vi "Manual_control.vi"(3 "Movement 2":T1={"Achsen-Wahl (X)"=36, "Richtung (vEw)"=0, "Geschwindigkeit\nin mm/s (5)[0,025-20]"=5.0, "IV6"=FALSE} {"Richtung (vEw)" items=["vom Endschalter weg", "zum Endschalter hin"]; "Geschwindigkeit\nin mm/s (5)[0,025-20]" min=0.025 max=20; "Achsen-Wahl (X)" items=["X-Achse"=36, "Y-Achse"=37, "Z-Achse"=38, "U-Achse"=63]}, 4 "Movement":T1={"Achsen-Wahl (X)"=36, "Richtung (vEw)"=0, "Geschwindigkeit\nin mm/s (5)[0,025-20]"=5.0, "IV6"=FALSE} {"Richtung (vEw)" items=["vom Endschalter weg", "zum Endschalter hin"]; "Geschwindigkeit\nin mm/s (5)[0,025-20]" min=0.025 max=20; "Achsen-Wahl (X)" items=["X-Achse"=36, "Y-Achse"=37, "Z-Achse"=38, "U-Achse"=63]}, 5 "error IO":errorcluster, 6 "Port for KOSY3":refnum<visa-resource-name>) -> (0 "Cordinates of the  KOSY3 Platform":T2 {"Schritte B" format="%#.4g"; "Schritte A" format="%#.4g"; "Schritte C" format="%#.4g"; "Schritte U" format="%#.4g"; "Schritte Z" format="%#.4g"; "Schritte Y" format="%#.4g"; "Schritte X" format="%#.4g"}, 1 "error out":errorcluster, 2 "VISA resource name out":refnum<visa-resource-name>)   [LabVIEW 2013]
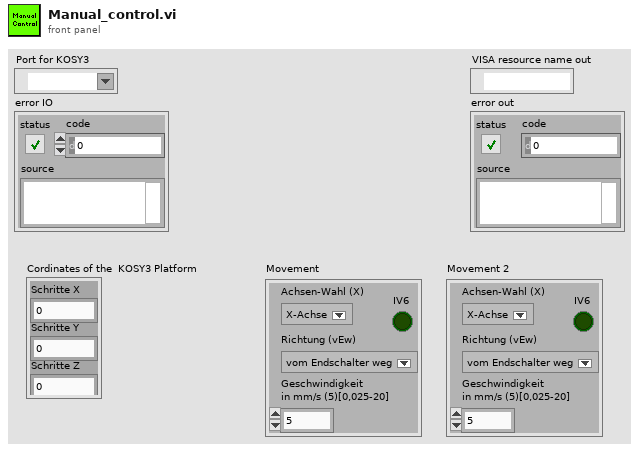
[diagram p1: front panel]
types:
  T1 = cluster{"Achsen-Wahl (X)":u8, "Richtung (vEw)":u8, "Geschwindigkeit\nin mm/s (5)[0,025-20]":sgl, "IV6":bool}
  T2 = cluster{"Schritte X":sgl, "Schritte Y":sgl, "Schritte Z":sgl, "Schritte U":sgl, "Schritte C":sgl, "Schritte A":sgl, "Schritte B":sgl}
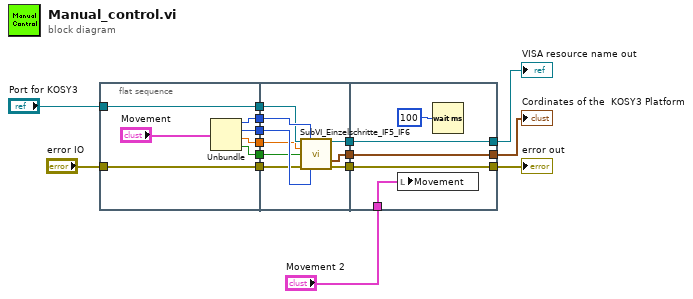
[diagram p0: block diagram]
diagram:
  n1 = flat-sequence {
    tunnel: [w22] -> w15
    tunnel: [w21] -> w14
    tunnel: [w20] -> w13
    tunnel: [w19] -> w12
    tunnel: [w18] -> w11
    tunnel: [w17] -> w10
    tunnel: "Port for KOSY3" -> [w18]
    tunnel: "error IO" -> [w17]
    tunnel: w15 -> [w30]
    tunnel: w14 -> [w23]
    tunnel: w13 -> [w31]
    tunnel: w12 -> [w28]
    tunnel: [w27] -> w9
    tunnel: [w29] -> w8
    tunnel: w11 -> [w26]
    tunnel: w10 -> [w25]
    tunnel: [w24] -> w7
    tunnel: w9 -> [w36]
    tunnel: w8 -> [w33]
    tunnel: w7 -> [w34]
    tunnel: [w33] -> w2
    tunnel: [w36] -> w3
    tunnel: [w34] -> w4
    tunnel: "Movement 2" -> [w32]
    frame #0 {
      n2 = Unbundle("Movement") -> ("Achsen-Wahl (X)"=w22:u8, "Richtung (vEw)"=w20:u8, "Geschwindigkeit\nin mm/s (5)[0,025-20]"=w21:sgl, "IV6"=w19:bool)
    }
    frame #1 {
      n3 = call "SubVI_Einzelschritte_IF5_IF6.vi"("VISA resource name in"=w26, "Achsen-Wahl (X)"=w30, "Geschwindigkeit\nin mm/s (5)[0,025-20]"=w23, "IF5=F/IF6=T\n(IF6=T) in"=w28, "error in"=w25, "Richtung (vEw)"=w31) -> ("VISA resource name out"=w24:refnum<visa-resource-name>, "Koordinaten IF6"=w29:T2, "error out"=w27:errorcluster)  [unwired: 3 in, 4 out]
    }
    frame #2 {
      n4 = local write "Movement"(w32) -> ()
      n5 = Wait (ms)(milliseconds to wait=u32 100) -> ()  [unwired: 1 out]
    }
  }
  "Cordinates of the  KOSY3 Platform" <- w2
  "VISA resource name out" <- w4
  "error out" <- w3
